vi "Lockin SR810.vi"(8 "error in (no error)":errorcluster, 11 "Lockin SR830 in":refnum<class "Lockin SR830.lvclass">) -> (0 "error out":errorcluster, 3 "Lockin SR830 out":refnum<class "Lockin SR830.lvclass">)   [LabVIEW 2009, in "Lockin SR830.lvclass"]
uses:
  Lockin SR830.lvclass
  Lockin SR830.lvclass/Lockin SR830.ctl
  Global/GPIB Numbers.vi
  Utility Classes/Readable/Readable.lvclass
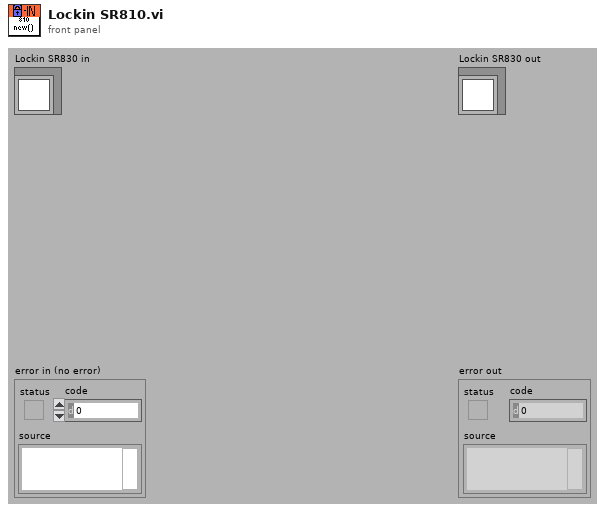
[diagram p1: front panel]
types:
  T1 = typedef "GPIB Type Def.ctl" = cluster{"Name":string, "bus":dbl, "GPIB":dbl, "GPIB as string":string, "byte":i32, "VISA Resource Name":refnum<visa-resource-name>}
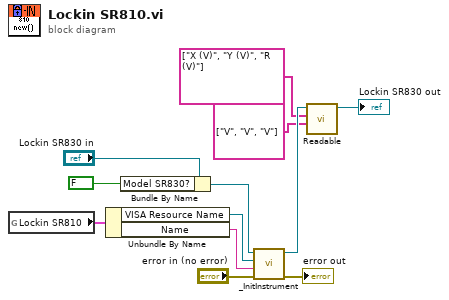
[diagram p0: block diagram]
diagram:
  n1 = global read "GPIB Numbers.vi" "Lockin SR810"() -> (w1:T1)
  n2 = Unbundle By Name(w1) -> ("VISA Resource Name"=w6:refnum<visa-resource-name>, "Name"=w7:string)
  n3 = Bundle By Name(cluster="Lockin SR830 in", "Model SR830?"=FALSE) -> (w11:refnum<class "Lockin SR830.lvclass">)
  n4 = call-dynamic "_InitInstrument.vi"("error in (no error)"="error in (no error)", "Name"=w7, "VISA Resource Name"=w6, "Instrument in"=w11) -> ("error out"=→"error out":errorcluster, "Instrument out"=w10:refnum<class "Lockin SR830.lvclass">)  [unwired: 2 in, 4 out]
  n5 = call "Readable.vi"("Channel Units"=string[] ["V", "V", "V"], "Channel Names"=string[] ["X (V)", "Y (V)", "R (V)"], "Readable in"=w10) -> ("Readable out"=→"Lockin SR830 out":refnum<class "Lockin SR830.lvclass">)  [unwired: 7 in, 1 out]
